vi "Filter_main_subvi.vi"(4 "Filter Order":i16, 6 "Filter Select":u16, 7 "Numeric in":dbl, 9 "Low Cut Off":dbl, 10 "High Cut Off":dbl, 11 "Filter or not":bool) -> (3 "Numeric out":dbl)   [LabVIEW 2020]
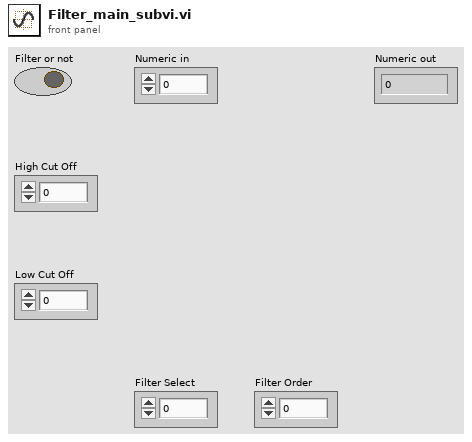
[diagram p1: front panel]
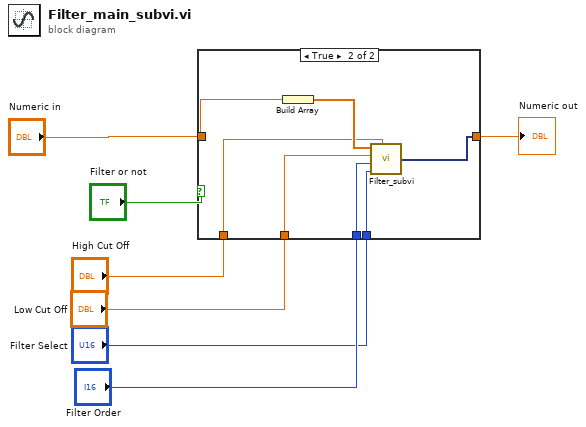
[diagram p0: block diagram]
diagram:
  n1 = case shown="True" "Filter or not" {
    tunnel: "Numeric in" -> [w8 w15]
    tunnel: [w8 w14] -> w1
    tunnel: "Filter Select" -> [_ w12]
    tunnel: "High Cut Off" -> [_ w11]
    tunnel: "Low Cut Off" -> [_ w10]
    tunnel: "Filter Order" -> [_ w9]
    frame False {
    }
    frame True {
      n2 = Build Array(w15) -> (w13:dbl[])
      n3 = call "Filter_subvi.vi"("Waveform"=w13, "Low Cut Off Frequency"=w10, "Filter Order"=w9, "Filter Select"=w12, "High Cut Off Frequency"=w11) -> ("Filtered Signal"=w14:dynamicdata)
    }
  }
  "Numeric out" <- w1
